vi "pressures.vi"() -> ()   [LabVIEW 2018]
uses:
  <vilib>/addons/h5labview2/file/H5Fmode.ctl
  <vilib>/addons/h5labview2/file/H5F.lvlib
  <vilib>/addons/h5labview2/group/H5G.lvlib
  <vilib>/addons/h5labview2/dataset/H5D.lvlib
panel:
  out "Chamber pressure (mbar)":cluster{"Chamber (mbar)":dbl}(graph)={"Chamber (mbar)"=0.00097618}
  in  "base name":string="pressure_"
  in  "Directory path":path=path "H:/data/pressure_data/20241011"
  out "Back pressure (mbar)":cluster{"Chamber (mbar)":dbl}(graph)={"Chamber (mbar)"=0.00097618}
  out "Chamber (mbar)":dbl=7.821100000000001e-08 format="%#_3e"
  out "Back (mbar)":dbl=0.00097618 format="%#_3e"
  in  "stop":bool
  # "Turbo Pump"
  # "Scroll (Roughing) Pump"
  # "Pump"
  # "Back\nPressure\nReadout"
  # "Gate"
  # "Roughing"
  # "Chamber\nPressure\nReadout"
  # "Chamber"
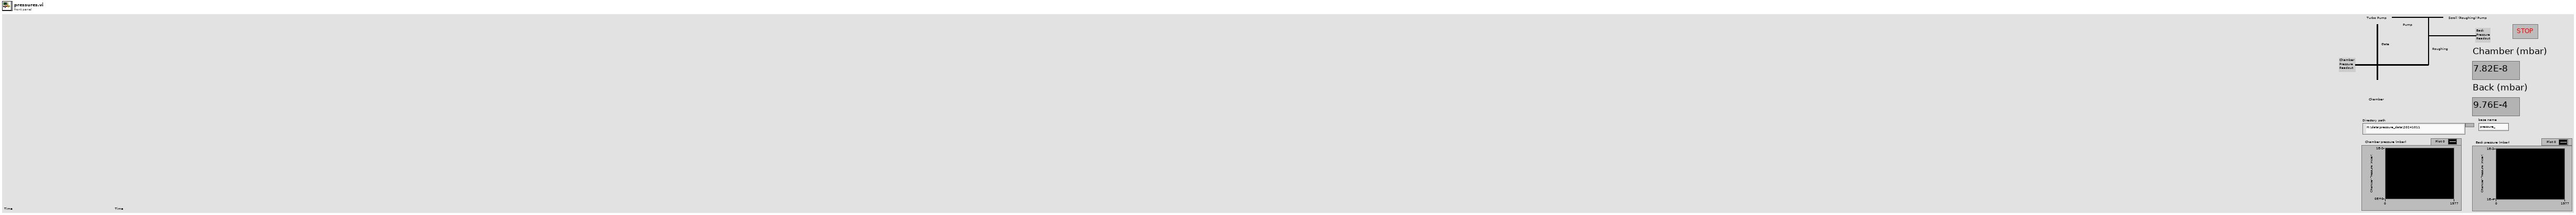
[diagram p1: front panel]
types:
  T1 = typedef "H5F.lvlib/H5Fmode.ctl" = enum16{"read-only", "read-write", "overwrite", "create new", "open or create"}
  T2 = typedef "hid_t.ctl" = i32
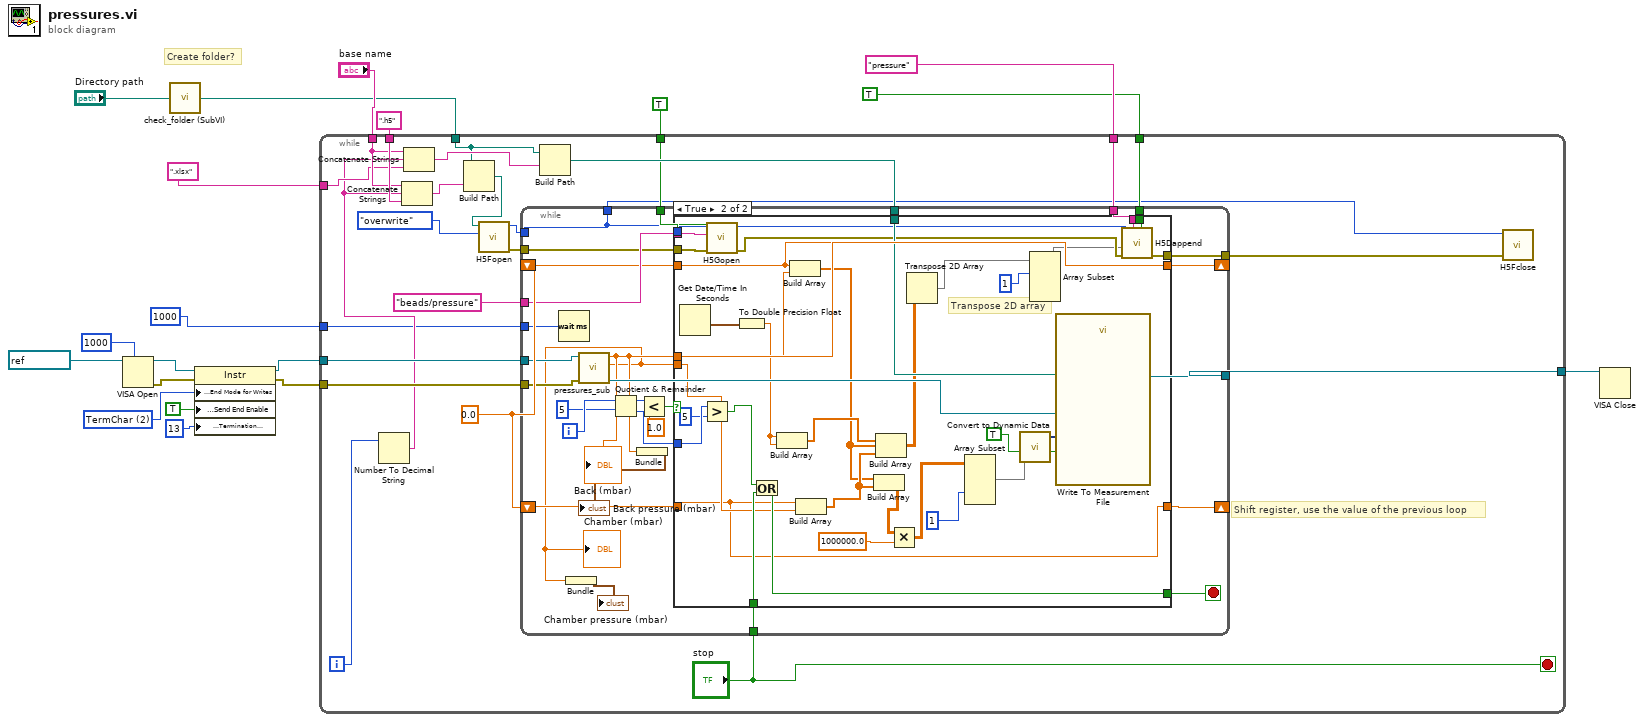
[diagram p0: block diagram]
diagram:
  w19 = u16 2 items=["None", "Last Bit", "TermChar", "Break"] ("Serial Settings:End Mode for Writes")
  # "Create folder?"
  n1 = VISA Open(timeout (0)=u32 1000 ("VISA Open timeout (0)"), VISA resource name=refnum<visa-resource-name> "COM7") -> (VISA resource name=w14:refnum<visa-resource-name>, error out=w11:errorcluster)  [unwired: 3 in]
  n2 = call "check_folder (SubVI).vi"("path in"="Directory path") -> ("path out"=w7:path)
  n3 = property class="Instr"(reference=w14, error in=w11, "Serial Settings:End Mode for Writes"=w19, "Message Based Settings:Send End Enable"=TRUE, "Message Based Settings:Termination Character"=u8 13) -> (reference out=w16:refnum<visa-resource-name>, error out=w12:errorcluster)
  n4 = while {
    tunnel: w16 -> [w44]
    tunnel: w12 -> [w43]
    tunnel: "base name" -> [w38]
    tunnel: ".h5" ("string") -> [w39]
    tunnel: w7 -> [w36]
    tunnel: ".xlsx" ("string") -> [w34]
    tunnel: u32 1000 ("milliseconds to wait") -> [w32]
    tunnel: [w31] -> w4
    tunnel: "pressure" ("dataset name") -> [w28]
    tunnel: TRUE ("replace? (F)") -> [w27]
    tunnel: TRUE ("create? (F)") -> [w25]
    i -> [w40]
    stop <- "stop" stop-if-true
    w26 = 0.0 ("Chamber (mbar)")
    # "Shift register, use the value of the previous loop"
    n5 = Number To Decimal String(number=w40) -> (decimal integer string=w33:string)  [unwired: 1 in]
    n6 = Concatenate Strings(w38, w33, w39) -> (w41:string)
    n7 = Concatenate Strings(w38, w33, w34) -> (w37:string)
    n8 = Build Path(base path=w36, name or relative path=w41) -> (appended path=w23:path)
    n9 = call <vilib>:"H5Fopen.vi"("mode (read-only)"=H5Fmode."overwrite", "path"=w23) -> ("error out"=w22:errorcluster, "ref out"=w21:T2)  [unwired: 8 in]
    n10 = Build Path(base path=w36, name or relative path=w37) -> (appended path=w35:path)
    n11 = while {
      tunnel: w44 -> [w71]
      tunnel: [w70] -> w31
      tunnel: w43 -> [w69]
      tunnel: w35 -> [w67]
      tunnel: "beads/pressure" ("name") -> [w66]
      tunnel: w32 -> [w65]
      tunnel: "stop" -> [w64]
      tunnel: [w62] -> w29
      tunnel: w28 -> [w61]
      tunnel: w27 -> [w60]
      shift-right: [w59] -> _
      shift-left: w26 -> [w58]
      shift-right: [w51] -> _
      shift-left: w26 -> [w57]
      tunnel: w25 -> [w56]
      tunnel: w22 -> [w55]
      tunnel: w21 -> [w54]
      tunnel: [w54] -> w20
      i -> [w50]
      stop <- w63 stop-if-true
      n12 = Wait (ms)(milliseconds to wait=w65) -> ()  [unwired: 1 out]
      n13 = call "pressures_sub.vi"("error in (no error)"=w69, "VISA Session In"=w71) -> ("VISA Session (Dup) Gauge1"=w70:refnum<visa-resource-name>, "Chamber (mbar)"=w52:dbl, "Back (mbar)"=w59:dbl)  [unwired: 7 in]
      "Back (mbar)" <- w59
      "Chamber (mbar)" <- w52
      n14 = Bundle("Chamber (mbar)"=w52) -> (→"Chamber pressure (mbar)":cluster{"Chamber (mbar)":dbl})  [unwired: 1 in]
      n15 = Quotient & Remainder(x=w50, y=5) -> (x-y*floor(x/y)=w47:i32, floor(x/y)=w45:i32)
      n16 = Bundle("Back (mbar)"=w59) -> (→"Back pressure (mbar)":cluster{"Back (mbar)":dbl})  [unwired: 1 in]
      n17 = Less?(x=w47, y=1.0) -> (x < y?=w46:bool)
      n18 = case shown="True" w46 {
        tunnel: w67 -> [_ w110]
        tunnel: w66 -> [_ w109]
        tunnel: w64 -> [w72 w108]
        tunnel: [w72 w107] -> w63
        tunnel: [w75 w104] -> w62
        tunnel: w61 -> [_ w103]
        tunnel: w60 -> [_ w102]
        tunnel: w59 -> [_ w100]
        tunnel: w58 -> [w74 w80]
        tunnel: w57 -> [w73 w79]
        tunnel: w56 -> [_ w84]
        tunnel: w55 -> [w75 w83]
        tunnel: w54 -> [_ w82]
        tunnel: w52 -> [_ w81]
        tunnel: [w74 w80] -> _
        tunnel: [w73 w79] -> w51
        tunnel: w45 -> [_ w77]
        frame False {
        }
        frame True {
          # "Transpose 2D array"
          n19 = Get Date/Time In Seconds() -> (seconds since 1Jan1904=w97:timestamp)
          n20 = Greater?(x=w77, y=5) -> (0:w78:bool)
          n21 = call <vilib>:"H5Gopen.vi"("create? (F)"=w84, "error in (no error)"=w83, "name"=w109, "ref in"=w82) -> ("error out"=w106:errorcluster, "group out"=w105:T2)  [unwired: 6 in]
          n22 = To Double Precision Float(number=w97) -> (double precision float=w96:dbl)
          n23 = Or(x=w78, y=w108) -> (x .or. y?=w107:bool)
          n24 = Build Array(w96, w96) -> (w94:dbl[])
          n25 = Build Array(w80, w100) -> (w88:dbl[])
          n26 = Build Array(w79, w81) -> (w93:dbl[])
          n27 = Build Array(w88, w93) -> (w89:dbl[][])
          n28 = Build Array(w94, w88, w93) -> (w101:dbl[][])
          n29 = Multiply(x=w89, y=1000000.0) -> (x*y=w86:dbl[][])
          n30 = Transpose 2D Array(2D array=w101) -> (transposed array=w99:dbl[][])
          n31 = Array Subset(array=w86, index (col)=1 ("index")) -> (w92:dbl[][])  [unwired: 3 in]
          n32 = call "Convert to Dynamic Data"("2D Array"=w92) -> ("Dynamic Data Type"=w91:dynamicdata)  [unwired: 3 in]
          n33 = Array Subset(array=w99, index (row)=1 ("index")) -> (w95:dbl[][])  [unwired: 3 in]
          n34 = call "Write To Measurement File"("Signals"=w91, "Flush? (T)"=TRUE, "Filename"=w110) -> ()  [unwired: 14 in, 3 out]
          n35 = call <vilib>:"H5Dappend.vi"("create? (T)"=w102, "dataset name"=w103, "error in (no error)"=w106, "data"=w95, "ref in"=w105) -> ("error out"=w104:errorcluster)  [unwired: 3 in, 3 out]
        }
      }
    }
    n36 = call <vilib>:"H5Fclose.vi"("error in (no error)"=w29, "ref"=w20) -> ()  [unwired: 9 in, 1 out]
  }
  n37 = VISA Close(VISA resource name=w4) -> ()  [unwired: 1 in, 1 out]
